vi "360.vi"   [LabVIEW 2017]
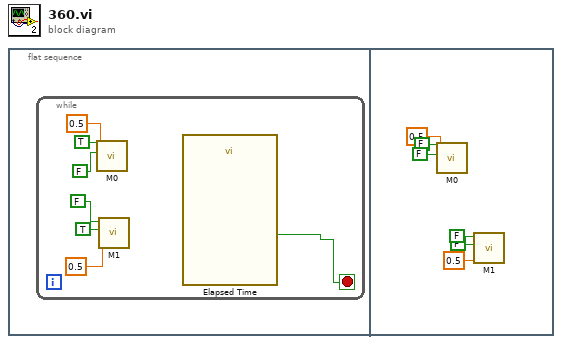
[diagram p0: block diagram]
diagram:
  n1 = flat-sequence {
    frame #0 {
      n2 = while {
        stop <- w1 stop-if-true
        n3 = call "M0.vi"("Duty Cycle"=0.5, "вперед"=FALSE, "назад"=TRUE) -> ()  [unwired: 8 in, 1 out]
        n4 = call "M1.vi"("Duty Cycle"=0.5, "вперед"=TRUE, "назад"=FALSE) -> ()  [unwired: 8 in, 1 out]
        n5 = call "Elapsed Time"() -> ("Time has Elapsed"=w1:bool)  [unwired: 12 in, 7 out]
      }
    }
    frame #1 {
      n6 = call "M0.vi"("Duty Cycle"=0.5, "вперед"=FALSE, "назад"=FALSE) -> ()  [unwired: 8 in, 1 out]
      n7 = call "M1.vi"("Duty Cycle"=0.5, "вперед"=FALSE, "назад"=FALSE) -> ()  [unwired: 8 in, 1 out]
    }
  }
